vi "T2.vi"() -> ()   [LabVIEW 2020]
panel:
  out "Este par?":bool
  in  "Numar":dbl
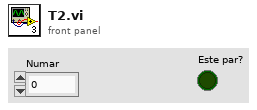
[diagram p1: front panel]
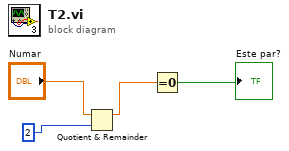
[diagram p0: block diagram]
diagram:
  n1 = Quotient & Remainder(x="Numar", y=2) -> (x-y*floor(x/y)=w1:dbl)  [unwired: 1 out]
  n2 = Equal To 0?(x=w1) -> (x = 0?=→"Este par?":bool)
